vi "3. Incorrect usage collections.vi"() -> ()   [LabVIEW 2017]
doc: "### Overview\n\nDemonstrates incorrect API String descriptions.\n\n### Instruction\n\nSelect **Action**, run the VI, and view the results. Incorrect formats will result in converted data that does not match the expected data.\n\n### Introduction\n\nThis example focuses especially on the Cluster data type, due to its complexity. Generally, the description format for Cluster data types falls into two categories:\n\n1. Tag:Value Mode\n2. No-Tag Mode\n\nThis example demonstrates some instances of incorrect API String descriptions."
uses:
  8f60ddcf-0cb1-4fc8-acc6-41852b9c13b8.vi
  addons/API-String-Arugments-Support/_Support/Convert API String Arguments to Data(variant).vi
panel:
  in  "Action":T1(ring)
  out "Retrieved Process":T2={"Expected Results"={"Child"=["a", "b", "c"], "Name"="csm", "Bool"=FALSE}, "String"="[a,b,c];Name: csm", "Reference Cluster"={"Child"=[], "Name"="", "Bool"=FALSE}, "Equal?"=FALSE, "Retrieved Data"={"Child"=["a", "b", "c"], "Name"="Name: csm", "Bool"=FALSE}}
  # "#CSM-Example Overview\n\nDemonstrates incorrect API String descriptions."
  # "#CSM-Example Instruction\n\nSelect **Action**, run the VI, and view the results. Incorrect formats will result in converted data that does not match the expected data."
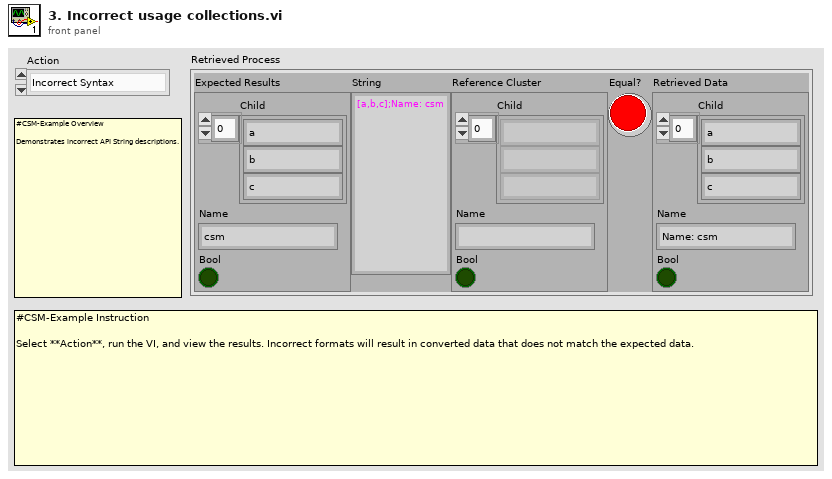
[diagram p1: front panel]
types:
  T1 = enum16{"Incorrect Syntax", "Correct Syntax 1", "Correct Syntax 2"}
  T2 = cluster{"Expected Results":cluster{"Child":string[], "Name":string, "Bool":bool}, "String":string, "Reference Cluster":cluster{"Child":string[], "Name":string, "Bool":bool}, "Equal?":bool, "Retrieved Data":cluster{"Child":string[], "Name":string, "Bool":bool}}
  T3 = cluster{"Child":string[], "Name":string, "Bool":bool}
  T4 = cluster{"Expected Results":cluster{"Child":string[], "Name":string, "Bool":bool}, "String":string, "Reference Cluster":cluster{"Child":string[], "Name":string, "Bool":bool}, bool, "Data":cluster{"Child":string[], "Name":string, "Bool":bool}}
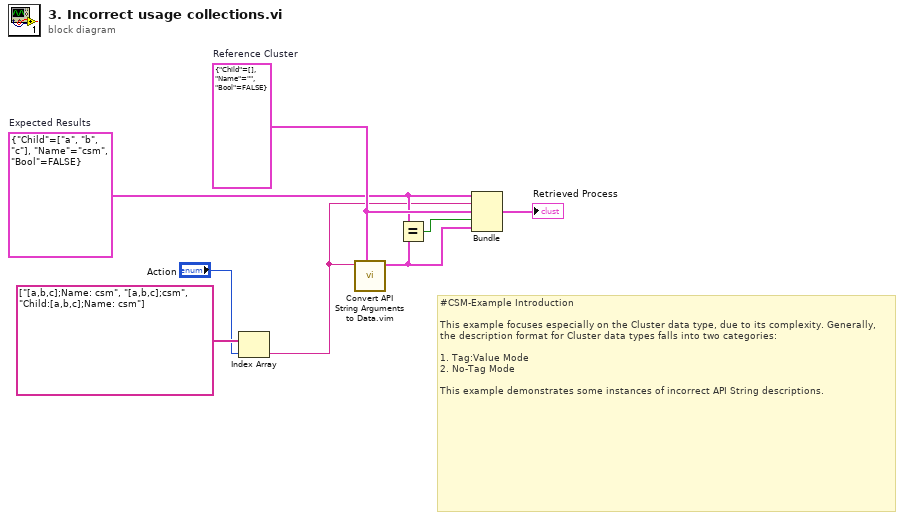
[diagram p0: block diagram]
diagram:
  w7 = T3 {"Child"=["a", "b", "c"], "Name"="csm", "Bool"=FALSE}  # Expected Results
  w8 = T3 {"Child"=[], "Name"="", "Bool"=FALSE}  # Reference Cluster
  # "#CSM-Example Introduction\n\nThis example focuses especially on the Cluster data type, due to its complexity. Generally, the description format for Cluster data types falls into two categories:\n\n1. Tag:Value Mode\n2. No-Tag Mode\n\nThis example demonstrates some instances of incorrect API String descriptions."
  n1 = Index Array(array=string[] ["[a,b,c];Name: csm", "[a,b,c];csm", "Child:[a,b,c];Name: csm"] ("String"), index="Action") -> (element=w1:string)
  n2 = call "Convert API String Arguments to Data.vim"("Reference Type"=w8, "API String"=w1) -> ("Data"=w5:T3)  [unwired: 6 in, 1 out]
  n3 = Equal?(x=w7, y=w5) -> (x = y?=w6:bool)
  n4 = Bundle("Expected Results"=w7, "String"=w1, "Reference Cluster"=w8, w6, "Data"=w5) -> (→"Retrieved Process":T4)  [unwired: 1 in]
